vi "Select First Item.vi"(8 "error in (no error)":errorcluster, 11 "Application Data in":T1) -> (0 "error out":errorcluster, 3 "Application Data out":T1)   [LabVIEW 2017, in "DSF Core.lvlib"]
uses:
  DSF Core.lvlib
  Main VI/Application Data.ctl
  <vilib>/NI/Memory Manager/Classes/Pointer/Pointer.lvclass
  Classes/Framework/Framework.lvclass
  Buffer Reader/Buffer Data.ctl
  Classes/Buffer/Buffer.lvclass
  Classes/Transfer Group Status/Status.lvclass
  Typedefs/DSF Data Type.ctl
  Typedefs/DSF Engine Channel Configuration.ctl
  Typedefs/DSF Settings Info.ctl
  Typedefs/DSF Byte Order.ctl
  Typedefs/DSF Engine Framework Configuration.ctl
  Typedefs/DSF Engine Plugin Configuration.ctl
  Typedefs/DSF Timing Info.ctl
  Typedefs/DSF Engine Plugin Thread Configuration.ctl
  Typedefs/DSF Engine Transfer Group Configuration.ctl
  Typedefs/DSF Direction.ctl
  Typedefs/DSF Engine Transfer Configuration.ctl
  Typedefs/DSF Timeout Behavior.ctl
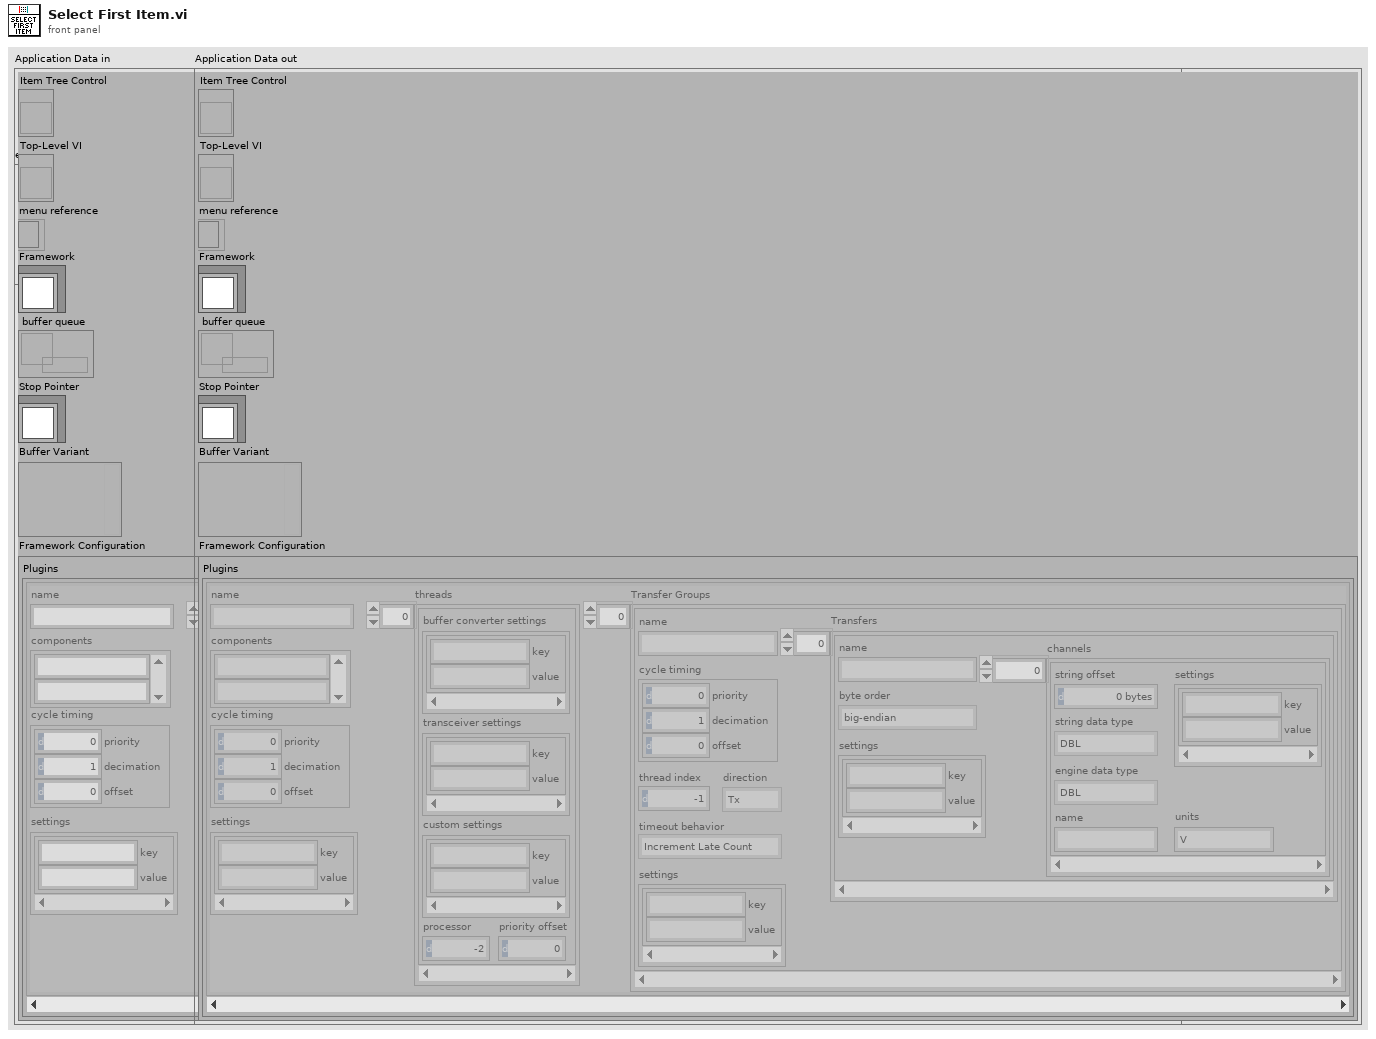
[diagram p1: front panel]
types:
  T1 = typedef "DSF Core.lvlib/Application Data.ctl" = cluster{"Item Tree Control":refnum<vi>, "Top-Level VI":refnum<vi>, "menu reference":refnum<k9>, "Framework":refnum<class "Framework.lvclass">, "buffer queue":refnum<queue>, "Stop Pointer":refnum<class "Pointer.lvclass">, "Buffer Variant":variant, "Framework Configuration":T2}
  T2 = typedef "DSF Core.lvlib/DSF Engine Framework Configuration.ctl" = cluster{"Plugins":T3[]}
  T3 = typedef "DSF Core.lvlib/DSF Engine Plugin Configuration.ctl" = cluster{"name":string, "components":string[], "cycle timing":T4, "threads":T5[], "Transfer Groups":T7[], "settings":T6}
  T4 = typedef "DSF Core.lvlib/DSF Timing Info.ctl" = cluster{"priority":u64, "decimation":u64, "offset":u64}
  T5 = typedef "DSF Core.lvlib/DSF Engine Plugin Thread Configuration.ctl" = cluster{"buffer converter settings":T6, "transceiver settings":T6, "custom settings":T6, "processor":i32, "priority offset":i16}
  T6 = typedef "DSF Core.lvlib/DSF Settings Info.ctl" = cluster{"key":string, "value":string}[]
  T7 = typedef "DSF Core.lvlib/DSF Engine Transfer Group Configuration.ctl" = cluster{"name":string, "direction":T8, "cycle timing":T4, "thread index":i32, "settings":T6, "Transfers":T9[], "timeout behavior":T13}
  T8 = typedef "DSF Core.lvlib/DSF Direction.ctl" = enum8{"Tx", "Rx"}
  T9 = typedef "DSF Core.lvlib/DSF Engine Transfer Configuration.ctl" = cluster{"name":string, "byte order":T10, "settings":T6, "channels":T11[]}
  T10 = typedef "DSF Core.lvlib/DSF Byte Order.ctl" = enum8{"big-endian", "little-endian"}
  T11 = typedef "DSF Core.lvlib/DSF Engine Channel Configuration.ctl" = cluster{"string offset":u64, "string data type":T12, "engine data type":T12, "name":string, "settings":T6, "units":string}
  T12 = typedef "DSF Core.lvlib/DSF Data Type.ctl" = enum8{"Bool", "SGL", "DBL", "I8", "I16", "I32", "I64", "U8", "U16", "U32", "U64"}
  T13 = typedef "DSF Core.lvlib/DSF Timeout Behavior.ctl" = enum8{"Increment Late Count", "Throw Error"}
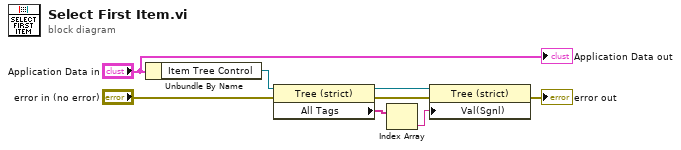
[diagram p0: block diagram]
diagram:
  n1 = Unbundle By Name("Application Data in") -> ("Item Tree Control"=w2:refnum<vi>)
  n2 = property class="Tree (strict)"(reference=w2, error in="error in (no error)") -> (reference out=w4:refnum<vi>, error out=w7:errorcluster, "All Tags"=w3:string[])
  n3 = Index Array(array=w3) -> (element=w5:string)  [unwired: 1 in]
  n4 = property class="Tree (strict)"(reference=w4, error in=w7, "Val(Sgnl)"=w5) -> (error out=→"error out":errorcluster)  [unwired: 1 out]
  "Application Data out" <- "Application Data in"
